vi "Spartan HTTP File Not Found Error Reply.vi"(4 "reply in":T2, 7 "env":T1) -> (0 "reply":T2, 3 "env out":T1)   [LabVIEW 2011]
uses:
  ITK EXT/http/cgi.llb/CGI Reply.ctl
  ITK EXT/utils/keyedarr.llb/Keyed Array.ctl
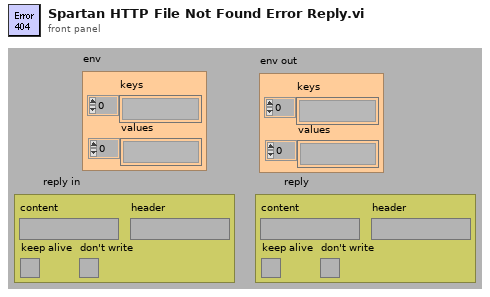
[diagram p1: front panel]
types:
  T1 = typedef "Keyed Array.ctl" = cluster{"keys":string[], "values":string[]}
  T2 = typedef "CGI Reply.ctl" = cluster{"content":string, "header":string, "keep alive":bool, "don't write":bool}
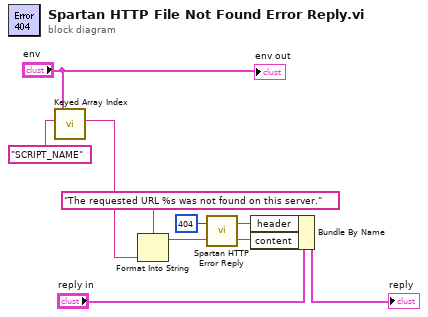
[diagram p0: block diagram]
diagram:
  n1 = call "Keyed Array Index.vi"("key"="SCRIPT_NAME" ("name"), "array in"="env") -> ("value"=w1:string)  [unwired: 2 in, 3 out]
  n2 = Format Into String(format string="The requested URL %s was not found on this server.", w1) -> (resulting string=w6:string)  [unwired: 2 in, 1 out]
  n3 = call "Spartan HTTP Error Reply.vi"("message"=w6, "status code"=404) -> ("content"=w9:string, "header"=w10:string)
  n4 = Bundle By Name(cluster="reply in", "header"=w10, "content"=w9) -> (→"reply":T2)
  "env out" <- "env"
